vi "Loop_HW.vi"() -> ()   [LabVIEW 2017, in "TemplateActuator.lvlib"]
uses:
  TemplateActuator.lvlib
  Globals/Global_STOP.vi
  Global_SM_Data Out.vi
  Global_HW_Data Out.vi
  Cluster_HW Status.ctl
  Cluster_SM To HW Data.ctl
panel:
  out "SM_Data In":T1
  out "HW Status":T2
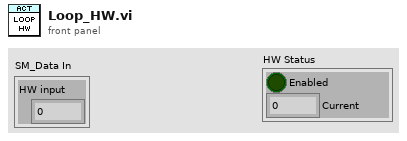
[diagram p1: front panel]
types:
  T1 = typedef "TemplateActuator.lvlib/Cluster_SM To HW Data.ctl" = cluster{"HW input":dbl}
  T2 = typedef "TemplateActuator.lvlib/Cluster_HW Status.ctl" = cluster{"Enabled":bool, "Current":dbl}
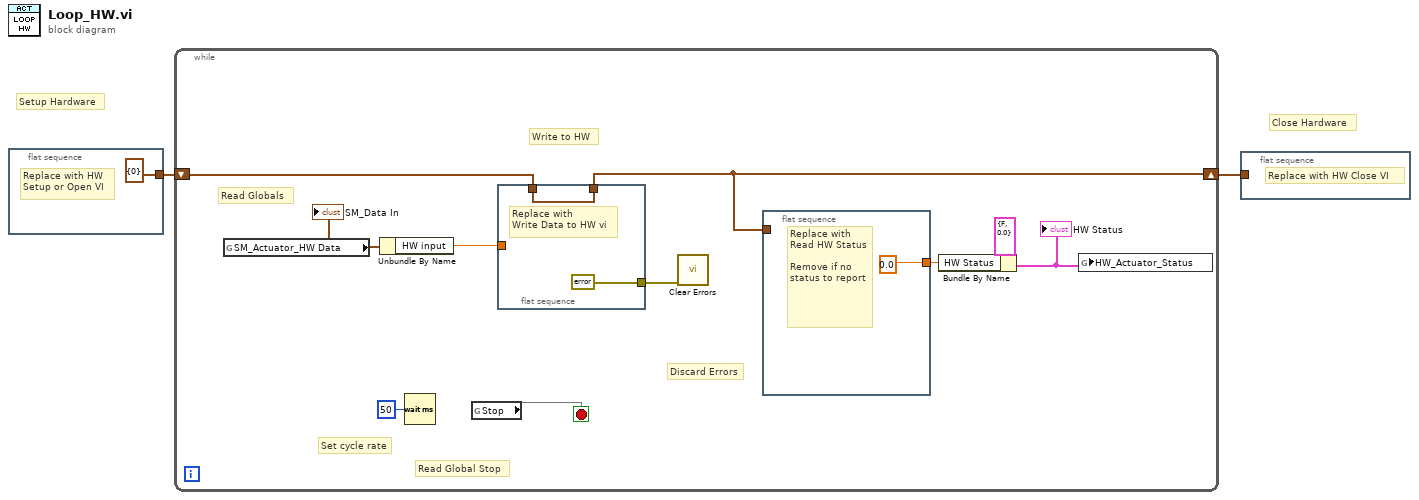
[diagram p0: block diagram]
diagram:
  # "Close Hardware"
  # "Setup Hardware"
  n1 = flat-sequence {
    tunnel: [cluster{i32} {0}] -> w2
    frame #0 {
      # "Replace with HW\nSetup or Open VI"
    }
  }
  n2 = while {
    shift-right: [w7] -> w1
    shift-left: w2 -> [w11]
    stop <- w13 stop-if-true
    # "Discard Errors"
    # "Write to HW"
    # "Read Globals"
    # "Read Global Stop"
    # "Set cycle rate"
    n3 = global read "Global_SM_Data Out.vi" "SM_Actuator_HW Data"() -> (w9:T1)
    "SM_Data In" <- w9
    n4 = Unbundle By Name(w9) -> ("HW input"=w8:dbl)
    n5 = Wait (ms)(milliseconds to wait=u32 50) -> ()  [unwired: 1 out]
    n6 = global read "Global_Stop.vi" "Stop"() -> (w13)
    n7 = flat-sequence {
      tunnel: w11 -> [w16]
      tunnel: [w16] -> w7
      tunnel: [errorcluster {"status"=FALSE, "code"=0, "source"=""} ("error constant")] -> w10
      tunnel: w8 -> [_]
      frame #0 {
        # "Replace with\nWrite Data to HW vi"
      }
    }
    n8 = call <vilib>:"Clear Errors.vi"("error in (no error)"=w10) -> ()  [unwired: 5 in, 2 out]
    n9 = flat-sequence {
      tunnel: w7 -> [_]
      tunnel: [0.0 ("HW Status")] -> w4
      frame #0 {
        # "Replace with Read HW Status\n\nRemove if no\nstatus to report"
      }
    }
    n10 = Bundle By Name(cluster=T2 {"Enabled"=FALSE, "Current"=0.0} ("HW_Actuator_Status"), "HW Status"=w4) -> (w5:T2)
    "HW Status" <- w5
    n11 = global write "Global_HW_Data Out.vi" "HW_Actuator_Status"(w5) -> ()
  }
  n12 = flat-sequence {
    tunnel: w1 -> [_]
    frame #0 {
      # "Replace with HW Close VI"
    }
  }
